vi "Create Image Type.vi"(8 "error in (no error)":errorcluster, 9 "Image Type":T2 items=["Grayscale (U8)", "Grayscale (I16)", "Grayscale (SGL)", "Complex (CSG)", "RGB (U32)", "HSL (U32)", "RGB (U64)", "Grayscale (U16)"], 10 "Image Name":string, 11 "Refnum in":T1) -> (0 "error out":errorcluster, 2 "Image Name (out)":string, 3 "Refnum out":T1)   [LabVIEW 2021, in "Image.lvlib"]
uses:
  <vilib>/vision/Image Controls.llb/IMAQ Image.ctl
  Image.lvlib
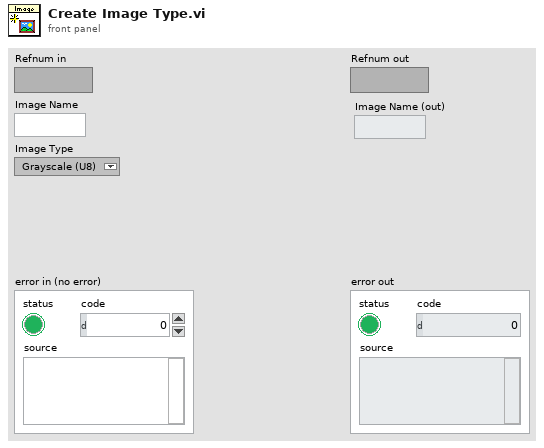
[diagram p1: front panel]
types:
  T1 = typedef "IMAQ Image.ctl" = refnum<image>
  T2 = typedef "Image Type" = u32
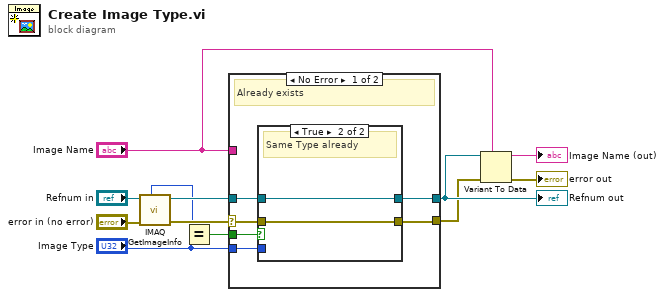
[diagram p0: block diagram]
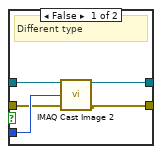
[diagram p2: hidden frame]
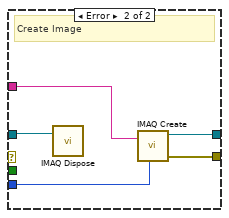
[diagram p3: hidden frame]
diagram:
  n1 = call "IMAQ GetImageInfo"("error in (no error)"="error in (no error)", "Image"="Refnum in") -> ("error out"=w11:errorcluster, "Image Type"=w7:T2)  [unwired: 2 in, 6 out]
  n2 = Equal?(x=w7, y="Image Type") -> (x = y?=w6:bool)
  n3 = case shown="No Error" w11 {
    selector: w11 -> [w14 _]
    tunnel: [w13 w28] -> w3
    tunnel: [w15 w26] -> w5
    tunnel: "Refnum in" -> [w16 w29]
    tunnel: "Image Name" -> [_ w27]
    tunnel: "Image Type" -> [w12 w25]
    tunnel: w6 -> [w17 _]
    frame No Error {
      # "Already exists"
      n4 = case shown="True" w17 {
        tunnel: w16 -> [w22 w24]
        tunnel: [w18 w24] -> w15
        tunnel: w14 -> [w20 w23]
        tunnel: [w19 w23] -> w13
        tunnel: w12 -> [w21 _]
        frame False {
          # "Different type"
          n5 = call "IMAQ Cast Image 2"("Image Src"=w22, "Image Type"=w21, "error in (no error)"=w20) -> ("Image Dst Out"=w18:T1, "error out"=w19:errorcluster)  [unwired: 11 in]
        }
        frame True {
          # "Same Type already"
        }
      }
    }
    frame Error {
      # "Create Image"
      n6 = call "IMAQ Dispose"("Image"=w29) -> ()  [unwired: 5 in, 1 out]
      n7 = call "IMAQ Create"("Image Name"=w27, "Image Type"=w25) -> ("New Image"=w26:T1, "error out"=w28:errorcluster)  [unwired: 3 in]
    }
  }
  "Refnum out" <- w5
  n8 = Variant To Data(error in=w3, type="Image Name", Variant=w5) -> (data=→"Image Name (out)":string, error out=→"error out":errorcluster)
